vi "Finalize To Settings.vi"(8 "error in (no error)":errorcluster, 11 "Core Groups Configuration in":refnum<class "Group Configuration.lvclass">) -> (0 "error out":errorcluster, 2 "settings":cluster{"key":string, "value":string}[](array[cluster]), 3 "Core Groups Configuration out":refnum<class "Group Configuration.lvclass">)   [LabVIEW 2021, in "DSF Core.lvlib" / "Group Configuration.lvclass"]
uses:
  Group Configuration.lvclass
  Group Configuration.lvclass/Group Configuration.ctl
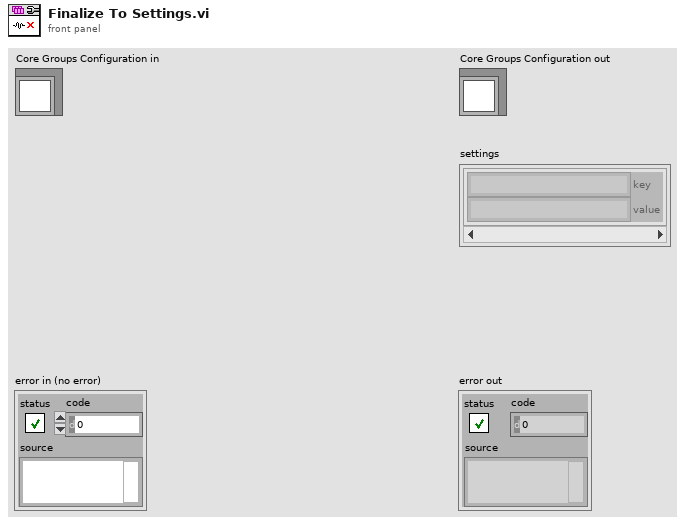
[diagram p1: front panel]
types:
  T1 = typedef "DSF Core.lvlib/Group Configuration.lvclass/Core Group Configuration.ctl" = cluster{"name":string, "direction":T2, "cycle timing":T3, "timeout behavior":T4, "enable conversion":bool}
  T2 = typedef "DSF Core.lvlib/DSF Direction.ctl" = enum8{"Tx", "Rx"}
  T3 = typedef "DSF Core.lvlib/DSF Timing Info.ctl" = cluster{"priority":u64, "decimation":u64, "offset":u64}
  T4 = typedef "DSF Core.lvlib/DSF Timeout Behavior.ctl" = enum8{"Increment Late Count", "Throw Error"}
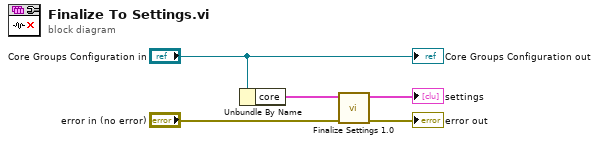
[diagram p0: block diagram]
diagram:
  n1 = Unbundle By Name("Core Groups Configuration in") -> ("core"=w3:T1)
  n2 = call "Finalize Settings 1.0.vi"("error in (no error)"="error in (no error)", "configuration 1.0"=w3) -> ("error out"=→"error out":errorcluster, "settings"=→"settings":cluster{"key":string, "value":string}[])  [unwired: 7 in, 1 out]
  "Core Groups Configuration out" <- "Core Groups Configuration in"
